vi "Stop Execution.vi"(1 "Stop":bool) -> (0 "Stop Dup":bool)   [LabVIEW 2020, in "FlexBlocks.lvlib"]
uses:
  FlexBlocks.lvlib
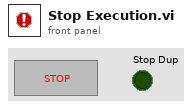
[diagram p1: front panel]
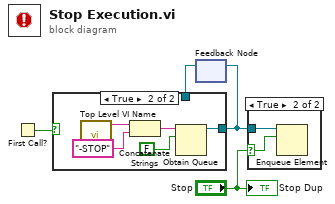
[diagram p0: block diagram]
diagram:
  n1 = First Call?() -> (First Call?: T/F=w4:bool)
  n2 = feedback #1() -> (w3:refnum<queue>)  [unwired: 1 in]
  n3 = case shown="True" w4 {
    tunnel: [w5 w6] -> w2
    tunnel: w3 -> [w5 _]
    frame False {
    }
    frame True {
      n4 = call "Top Level VI Name.vi"() -> ("Top Level VI Name"=w9:string)  [unwired: 11 in]
      n5 = Concatenate Strings(w9, "-STOP" ("string")) -> (w10:string)
      n6 = Obtain Queue(name (unnamed)=w10, element data type=FALSE) -> (queue out=w6:refnum<queue>)  [unwired: 3 in, 2 out]
    }
  }
  n7 = feedback-in #1(w2) -> ()
  n8 = case shown="True" "Stop" {
    selector: "Stop" -> [_ w11]
    tunnel: w2 -> [_ w12]
    frame False {
    }
    frame True {
      n9 = Enqueue Element(queue=w12, element=w11) -> ()  [unwired: 2 in, 3 out]
    }
  }
  "Stop Dup" <- "Stop"
